vi "Global 1.vi"() -> ()   [LabVIEW 2013]
panel:
  in  "Eye x position":dbl
  out "Camera ready":bool
  out "camera stop":bool
  out "Eye tracker busy":bool
  out "Start one trial":bool
  out "global stop":bool
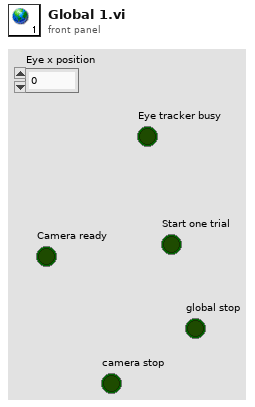
[diagram p1: front panel]
diagram:
